vi "lua_pushboolean.vi"(8 "error in (no error)":errorcluster, 10 "Boolean":bool, 11 "lua_state_p":u64) -> (0 "error out":errorcluster, 3 "lua_state_p out":u64)   [LabVIEW 2020, in "lua.dll.lvlib"]
uses:
  lua.dll.lvlib
  lua54.dll
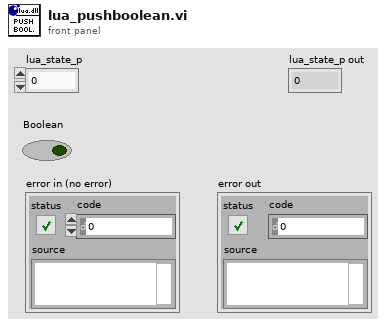
[diagram p1: front panel]
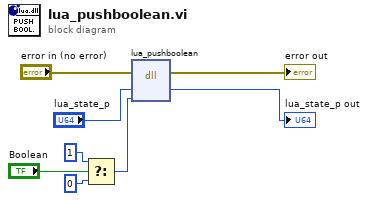
[diagram p0: block diagram]
diagram:
  n1 = Select(t=1 ("int"), s="Boolean", f=0 ("int")) -> (s? t:f=w1:i32)
  n2 = dll-call lib="C:/Users/Nicholas Folse/Documents/workspace/github-tauterra.llc/Lua for LabVIEW/lib/lua.dll/lua54**.*" fn="lua_pushboolean"(error in="error in (no error)", "lua_state_p"="lua_state_p", "int"=w1) -> (error out=→"error out":errorcluster, "lua_state_p"=→"lua_state_p out":u64)  [unwired: 4 in, 1 out]
